vi "Sequence Timeout 6301--error.vi"() -> (0 "error out":errorcluster)   [LabVIEW 2024, in "Auto Modo.lvlib"]
uses:
  Auto Modo.lvlib
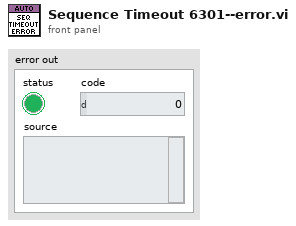
[diagram p1: front panel]
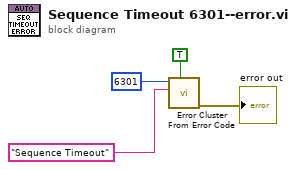
[diagram p0: block diagram]
diagram:
  n1 = call <vilib>:"Error Cluster From Error Code.vi"("show call chain? (False)"=TRUE, "error message (\"\")"="Sequence Timeout" ("error message (\"\")"), "error code (0)"=6301) -> ("error out"=→"error out":errorcluster)  [unwired: 6 in]
